vi "LIMITS.vi"(8 "Error In":errorcluster, 11 "User Creds":T1) -> (0 "Error Out":errorcluster, 2 "Bool Lims Out":T2, 3 "LIMITS Out":cluster{"LIMITS1-20":dbl[], "LIMITS21-40":dbl[]})   [LabVIEW 2023, in "QSM - Limits.lvlib"]
uses:
  Limits.ctl
  QSM - Limits/Controls/State Machine Message.ctl
  QSM - Limits/Controls/Message Queue Element Position.ctl
  QSM - Limits/QSM - Limits.lvlib
  QSM - Main/QSM - Main.lvlib
  UserCredentials.ctl
panel:
  in  "Bool Lims":T2
  in  "CLOSE":bool
  in  "SAVE":bool
  in  "LIMITS":T3
  # "--LIMITS--"
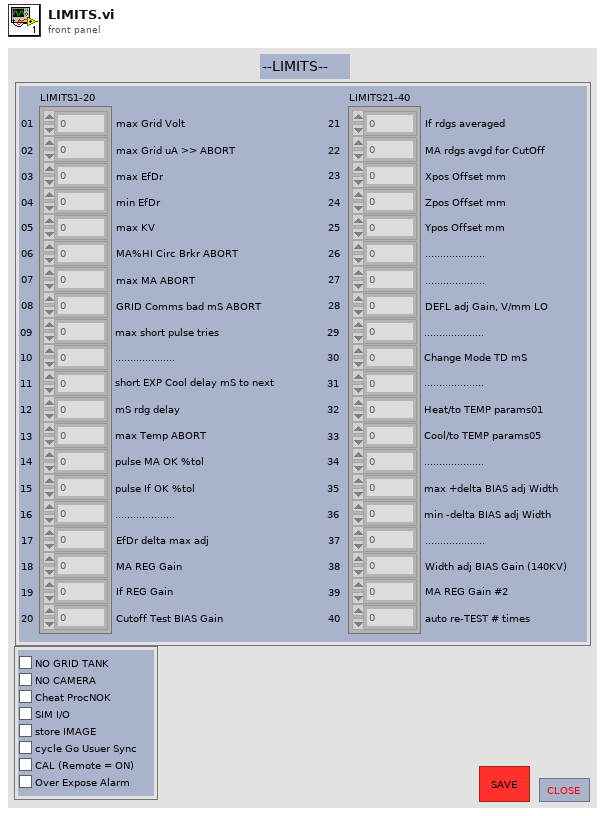
[diagram p1: front panel]
types:
  T1 = typedef "UserCredentials.ctl" = cluster{"Badge Number":string, "Name":string, "Access":enum16{"", "Operator", "Admin", "Engineer"}}
  T2 = cluster{"NO GRID TANK":bool, "NO GRID TANK 2":bool, "NO GRID TANK 3":bool, "NO GRID TANK 4":bool, "NO GRID TANK 5":bool, "NO GRID TANK 6":bool, "NO GRID TANK 7":bool, "NO GRID TANK 8":bool}
  T3 = typedef "Limits.ctl" = cluster{"LIMITS1-20":sgl[], "LIMITS21-40":sgl[]}
  T4 = typedef "QSM - Limits.lvlib/State Machine Message.ctl" = enum16{"Initialize", "SAVE Button", "Handle Error", "Exit"}
  T5 = typedef "QSM - Limits.lvlib/Message Queue Element Position.ctl" = enum16{"Front", "Back"}
  T6 = enum8{"Enabled", "Disabled", "Disabled and Grayed Out"}
  T7 = cluster{"Boolean array[0]":bool, "Boolean array[1]":bool, "Boolean array[2]":bool, "Boolean array[3]":bool, "Boolean array[4]":bool, "Boolean array[5]":bool, "Boolean array[6]":bool, "Boolean array[7]":bool}
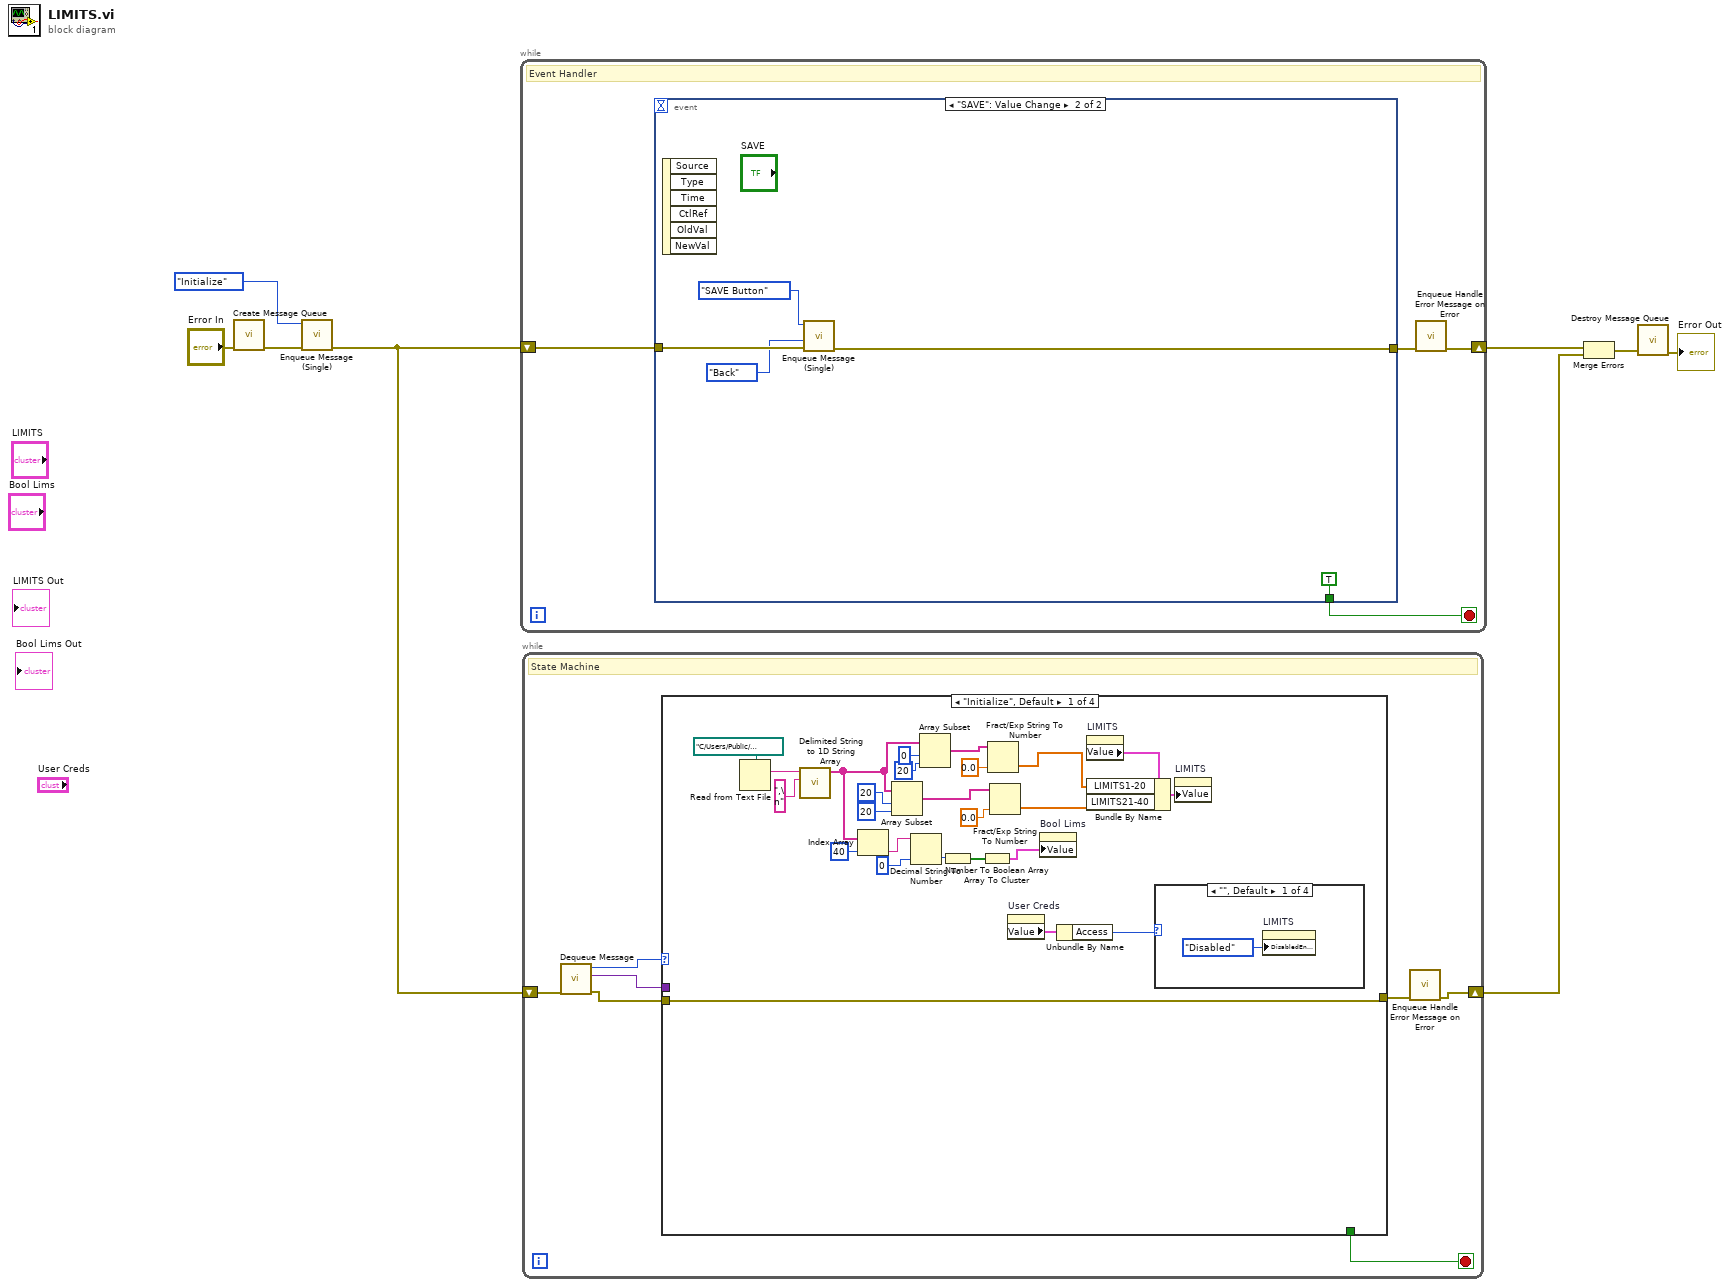
[diagram p0: block diagram]
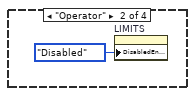
[diagram p2: hidden frame]
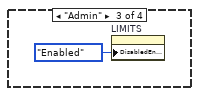
[diagram p3: hidden frame]
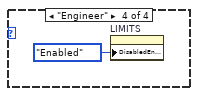
[diagram p4: hidden frame]
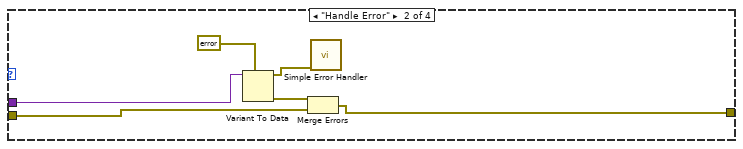
[diagram p5: hidden frame]
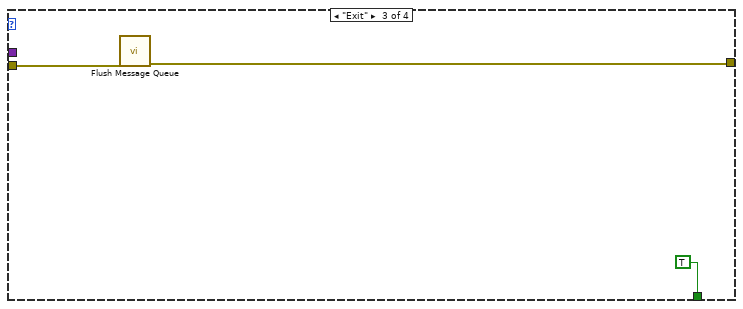
[diagram p6: hidden frame]
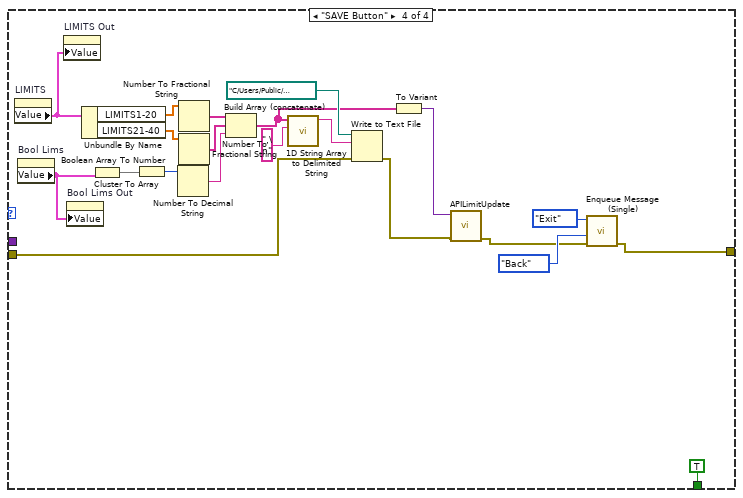
[diagram p7: hidden frame]
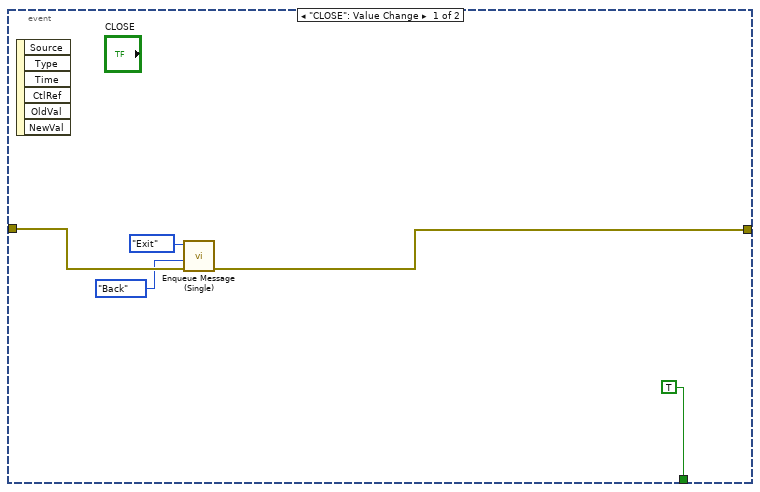
[diagram p8: hidden frame]
diagram:
  n1 = call "Create Message Queue.vi"("Error In"="Error In") -> ("Error Out"=w7:errorcluster)  [unwired: 10 in]
  n2 = call "Enqueue Message (Single).vi"("Error In"=w7, "State Machine Message"=State_Machine_Message."Initialize") -> ("Error Out"=w5:errorcluster)  [unwired: 9 in]
  n3 = while {
    shift-right: [w11] -> w3
    shift-left: w5 -> [w10]
    stop <- w9 stop-if-true
    # "Event Handler"
    n4 = event shown="[1] \"SAVE\": Value Change" {
      selector: _ -> [_ _]
      dyn-events: _ -> [_ _]
      timeout: _ -> [_ _]
      tunnel: [w14 w21] -> w12
      tunnel: w10 -> [w17 w22]
      tunnel: [TRUE TRUE] -> w9
      event "CLOSE": Value Change {
        n5 = event-data() -> ()  [unwired: 1 in, 6 out]
        n6 = call "Enqueue Message (Single).vi"("Error In"=w17, "Message Position"=Message_Queue_Element_Position."Back", "State Machine Message"=State_Machine_Message."Exit") -> ("Error Out"=w14:errorcluster)  [unwired: 8 in]
      }
      event "SAVE": Value Change {
        n7 = event-data() -> ()  [unwired: 1 in, 6 out]
        n8 = call "Enqueue Message (Single).vi"("Error In"=w22, "Message Position"=Message_Queue_Element_Position."Back", "State Machine Message"=State_Machine_Message."SAVE Button") -> ("Error Out"=w21:errorcluster)  [unwired: 8 in]
      }
    }
    n9 = call "Enqueue Handle Error Message on Error.vi"("Error In"=w12) -> ("Error Out"=w11:errorcluster)  [unwired: 10 in]
  }
  n10 = while {
    shift-right: [w25] -> w2
    shift-left: w5 -> [w29]
    stop <- w23 stop-if-true
    # "State Machine"
    n11 = call "Dequeue Message.vi"("Error In"=w29) -> ("Error Out"=w28:errorcluster, "Data"=w27:variant, "State Machine Message"=w26:T4)  [unwired: 8 in]
    n12 = case shown="\"Initialize\", Default" w26 {
      tunnel: w28 -> [w54 w61 w67 w75]
      tunnel: w27 -> [_ w59 _ _]
      tunnel: [w54 w60 w65 w76] -> w24
      tunnel: [_ _ TRUE TRUE] -> w23
      frame "Initialize", Default {
        n13 = Read from Text File(file (use dialog)=path "C:/Users/Public/Documents/Grid2093/LIMITS/LIMITS.txt") -> (text=w53:string)  [unwired: 3 in, 3 out]
        n14 = call <vilib>:"Delimited String to 1D String Array.vi"("delimiter"=",\n", "delimited string"=w53) -> ("string array"=w40:string[])  [unwired: 9 in]
        n15 = Index Array(array=w40, index=40) -> (element=w39:string)
        n16 = Array Subset(array=w40, index=20, length=20) -> (w43:string[])
        n17 = Decimal String To Number(string=w39, default (0L)=u32 0 ("default (0 I32)")) -> (number=w38:u32)  [unwired: 1 in, 1 out]
        n18 = Array Subset(array=w40, index=0, length=20) -> (w44:string[])
        n19 = Number To Boolean Array(number=w38) -> (Boolean array=w35:bool[])
        n20 = Array To Cluster(array=w35) -> (cluster=w34:T7)
        n21 = Fract/Exp String To Number(string=w44, default (0 dbl)=sgl 0.0 ("default (0 DBL)")) -> (number=w42:sgl[])  [unwired: 2 in, 1 out]
        n22 = Fract/Exp String To Number(string=w43, default (0 dbl)=sgl 0.0 ("default (0 DBL)")) -> (number=w41:sgl[])  [unwired: 2 in, 1 out]
        n23 = property on="User Creds" class="Clust (strict)"() -> ("Value"=w31:T1)  [unwired: 2 in, 2 out]
        n24 = property on="Bool Lims" class="Clust (strict)"("Value"=w34) -> ()  [unwired: 2 in, 2 out]
        n25 = Unbundle By Name(w31) -> ("Access"=w30:enum16{"", "Operator", "Admin", "Engineer"})
        n26 = property on="LIMITS" class="Clust (strict)"() -> ("Value"=w45:T3)  [unwired: 2 in, 2 out]
        n27 = Bundle By Name(cluster=w45, "LIMITS1-20"=w42, "LIMITS21-40"=w41) -> (w46:T3)
        n28 = case shown="\"\", Default" w30 {
          frame "", Default {
            n29 = property on="LIMITS" class="Clust (strict)"("DisabledEnum"=T6."Disabled" ("Disabled")) -> ()  [unwired: 2 in, 2 out]
          }
          frame "Operator" {
            n30 = property on="LIMITS" class="Clust (strict)"("DisabledEnum"=T6."Disabled" ("Disabled")) -> ()  [unwired: 2 in, 2 out]
          }
          frame "Admin" {
            n31 = property on="LIMITS" class="Clust (strict)"("DisabledEnum"=T6."Enabled" ("Disabled")) -> ()  [unwired: 2 in, 2 out]
          }
          frame "Engineer" {
            n32 = property on="LIMITS" class="Clust (strict)"("DisabledEnum"=T6."Enabled" ("Disabled")) -> ()  [unwired: 2 in, 2 out]
          }
        }
        n33 = property on="LIMITS" class="Clust (strict)"("Value"=w46) -> ()  [unwired: 2 in, 2 out]
      }
      frame "Handle Error" {
        n34 = Variant To Data(type=errorcluster {"status"=FALSE, "code"=0, "source"=""} ("Error In"), Variant=w59) -> (data=w62:errorcluster, error out=w63:errorcluster)  [unwired: 1 in]
        n35 = Merge Errors(w63, w61) -> (w60:errorcluster)
        n36 = call <vilib>:"Simple Error Handler.vi"("error in (no error)"=w62) -> ()  [unwired: 4 in, 5 out]
      }
      frame "Exit" {
        n37 = call "Flush Message Queue.vi"("Error In"=w67) -> ("Error Out"=w65:errorcluster)  [unwired: 9 in, 1 out]
      }
      frame "SAVE Button" {
        n38 = property on="LIMITS" class="Clust (strict)"() -> ("Value"=w73:T3)  [unwired: 2 in, 2 out]
        n39 = property on="Bool Lims" class="Clust (strict)"() -> ("Value"=w72:T2)  [unwired: 2 in, 2 out]
        n40 = property on="LIMITS Out" class="Clust (strict)"("Value"=w73) -> ()  [unwired: 2 in, 2 out]
        n41 = property on="Bool Lims Out" class="Clust (strict)"("Value"=w72) -> ()  [unwired: 2 in, 2 out]
        n42 = Unbundle By Name(w73) -> ("LIMITS1-20"=w88:sgl[], "LIMITS21-40"=w87:sgl[])
        n43 = Cluster To Array(cluster=w72) -> (array=w84:bool[])
        n44 = Boolean Array To Number(Boolean array=w84) -> (number=w83:u32)
        n45 = Number To Decimal String(number=w83) -> (decimal integer string=w82:string)  [unwired: 1 in]
        n46 = Number To Fractional String(number=w88) -> (F-format string=w86:string[])  [unwired: 3 in]
        n47 = Number To Fractional String(number=w87) -> (F-format string=w85:string[])  [unwired: 3 in]
        n48 = Build Array (concatenate)(w86, w85, w82) -> (w68:string[])
        n49 = call <vilib>:"1D String Array to Delimited String.vi"("delimiter"=",\n", "string array"=w68) -> ("delimited string"=w80:string)  [unwired: 9 in]
        n50 = Write to Text File(file (use dialog)=path "C:/Users/Public/Documents/Grid2093/LIMITS/LIMITS.txt", text=w80, error in=w75) -> (error out=w69:errorcluster)  [unwired: 1 in, 2 out]
        n51 = To Variant(anything=w68) -> (Variant=w71:variant)
        n52 = call "APILimitUpdate.vi"("Error In"=w69, "Data"=w71) -> ("Error Out"=w70:errorcluster)  [unwired: 9 in]
        n53 = call "Enqueue Message (Single).vi"("Error In"=w70, "Message Position"=Message_Queue_Element_Position."Back", "State Machine Message"=State_Machine_Message."Exit") -> ("Error Out"=w76:errorcluster)  [unwired: 8 in]
      }
    }
    n54 = call "Enqueue Handle Error Message on Error.vi"("Error In"=w24) -> ("Error Out"=w25:errorcluster)  [unwired: 10 in]
  }
  n55 = Merge Errors(w3, w2) -> (w4:errorcluster)
  n56 = call "Destroy Message Queue.vi"("Error In"=w4) -> ("Error Out"=→"Error Out":errorcluster)  [unwired: 10 in]
